vi "Controls Size Change.vi"(4 "서브패널 참조":refnum<vi>[](array[refnum]), 5 "선택된 기준기":refnum<vi>, 6 "탭 컨트롤":refnum<vi>, 7 "기준기 리스트":refnum<vi>, 8 "에러 입력(에러 없음)":errorcluster, 9 "교정절차 목록 List":refnum<vi>, 11 "출장교정 List":refnum<vi>) -> (0 "에러 출력":errorcluster)   [LabVIEW 2020]
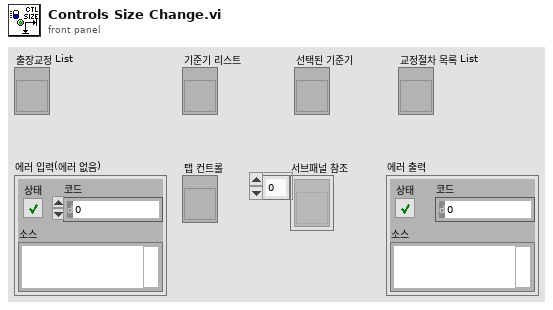
[diagram p1: front panel]
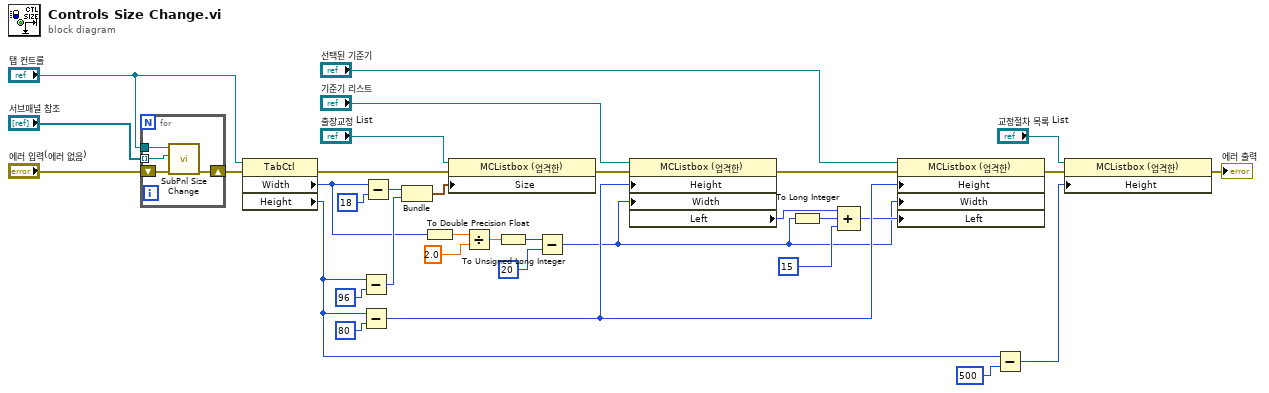
[diagram p0: block diagram]
diagram:
  n1 = for {
    tunnel: "탭 컨트롤" -> [w37]
    shift-right: [w36] -> w29
    shift-left: "에러 입력(에러 없음)" -> [w38]
    tunnel: "서브패널 참조" -> [w35] mode=indexing
    n2 = call "SubPnl Size Change.vi"("에러 입력(에러 없음)"=w38, "서브 패널"=w35, "TabControl 입력"=w37) -> ("에러 출력"=w36:errorcluster)  [unwired: 8 in]
  }
  n3 = property on="프로퍼티 노드" class="TabCtl"(reference="탭 컨트롤", error in=w29) -> (error out=w3:errorcluster, "Width"=w2:u32, "Height"=w1:u32)  [unwired: 1 out]
  n4 = Subtract(x=w1, y=u32 96) -> (x-y=w33:u32)
  n5 = Subtract(x=w1, y=u32 80) -> (x-y=w16:u32)
  n6 = Subtract(x=w2, y=u32 18) -> (x-y=w23:u32)
  n7 = Bundle(w23, w33) -> (w30:cluster{u32, u32})  [unwired: 1 in]
  n8 = To Double Precision Float(number=w2) -> (double precision float=w21:dbl)
  n9 = property on="프로퍼티 노드" class="MCListbox (엄격한)"(reference="출장교정 List", error in=w3, "Size"=w30) -> (error out=w24:errorcluster)  [unwired: 1 out]
  n10 = Divide(x=w21, y=2.0) -> (x/y=w20:dbl)
  n11 = To Unsigned Long Integer(number=w20) -> (unsigned 32bit integer=w15:u32)
  n12 = Subtract(x=w15, y=u32 20) -> (x-y=w10:u32)
  n13 = property class="MCListbox (엄격한)"(reference="기준기 리스트", error in=w24, "Height"=w16, "Width"=w10) -> (error out=w18:errorcluster, "Left"=w14:i32)  [unwired: 1 out]
  n14 = To Long Integer(number=w10) -> (32bit integer=w12:i32)
  n15 = Compound Arithmetic op=ADD(w14, w12, 15 ("값")) -> (w13:i32)
  n16 = property class="MCListbox (엄격한)"(reference="선택된 기준기", error in=w18, "Height"=w16, "Width"=w10, "Left"=w13) -> (error out=w8:errorcluster)  [unwired: 1 out]
  n17 = Subtract(x=w1, y=u32 500) -> (x-y=w4:u32)
  n18 = property class="MCListbox (엄격한)"(reference="교정절차 목록 List", error in=w8, "Height"=w4) -> (error out=→"에러 출력":errorcluster)  [unwired: 1 out]
